vi "XL320_Read U8 From 1 Address.vi"(8 "Error in (no error)":errorcluster, 9 "Address number (0)":u16 max=49, 10 "Motor ID (0)":u8, 11 "VISA resource name":refnum<visa-resource-name>) -> (0 "error out":errorcluster, 2 "Data":u8, 3 "VISA resource name out":refnum<visa-resource-name>)   [LabVIEW 2017, in "Dynamixel XL320.lvlib"]
doc: "Reads a single value/address from the motor's register. This is a Low-Level VI that is used by other VIs."
uses:
  <instrlib>/Dynamixel XL320 (Drivers instrument)/Dynamixel XL320.lvlib
panel:
  # "Ghislain REMY, IUT de Cachan, 2015 December 2015"
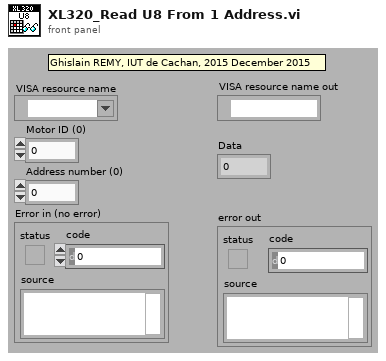
[diagram p1: front panel]
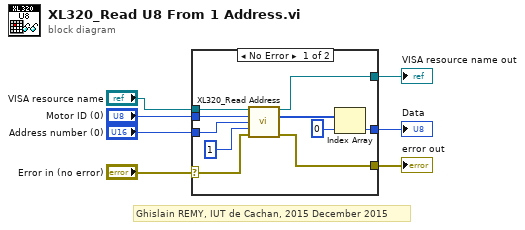
[diagram p0: block diagram]
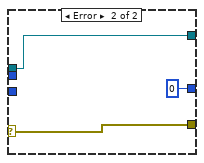
[diagram p2: hidden frame]
diagram:
  # "Ghislain REMY, IUT de Cachan, 2015 December 2015"
  n1 = case shown="No Error" "Error in (no error)" {
    selector: "Error in (no error)" -> [w11 w19]
    tunnel: [w17 u8 0 ("Numeric")] -> w7
    tunnel: "VISA resource name" -> [w15 w20]
    tunnel: [w8 w20] -> w5
    tunnel: [w10 w19] -> w4
    tunnel: "Motor ID (0)" -> [w14 _]
    tunnel: "Address number (0)" -> [w13 _]
    frame No Error {
      n2 = call <instrlib>:"XL320_Read Address.vi"("VISA resource name"=w15, "Motor ID (0)"=w14, "Address number (0)"=w13, "Number of Addresses to read (1)"=u16 1, "Error in (no error)"=w11) -> ("VISA resource name Out"=w8:refnum<visa-resource-name>, "Data Read"=w9:u8[], "error out"=w10:errorcluster)  [unwired: 7 in, 1 out]
      n3 = Index Array(array=w9, index=0) -> (element=w17:u8)
    }
    frame Error {
    }
  }
  "Data" <- w7
  "VISA resource name out" <- w5
  "error out" <- w4
